vi "Initialize.vi"(8 "error in (no error)":errorcluster, 9 "transceiver settings":T1, 10 "Transfer Groups Configurations":T2[](array[typedef]) {"Transfers"."channel configurations"."buffer offset" format="%d bytes"}, 11 "UDP Transceiver in":refnum<class "UDP Transceiver.lvclass">) -> (0 "error out":errorcluster, 3 "UDP Transceiver out":refnum<class "UDP Transceiver.lvclass">)   [LabVIEW 2017, in "UDP.lvlib" / "UDP Transceiver.lvclass"]
uses:
  UDP Transceiver.lvclass
  Builds/Data Sharing Framework/Current/Data Sharing Framework Core/DSF Core.lvlibp/Configuration/Public/Controls/DSF Engine Transfer Group Configuration.ctl
  Builds/Data Sharing Framework/Current/Data Sharing Framework Core/DSF Core.lvlibp/Configuration/Public/Controls/DSF Direction.ctl
  Builds/Data Sharing Framework/Current/Data Sharing Framework Core/DSF Core.lvlibp/Configuration/Public/Controls/DSF Timing Info.ctl
  Builds/Data Sharing Framework/Current/Data Sharing Framework Core/DSF Core.lvlibp/Configuration/Public/Controls/DSF Engine Transfer Configuration.ctl
  Builds/Data Sharing Framework/Current/Data Sharing Framework Core/DSF Core.lvlibp/Configuration/Public/Controls/DSF Byte Order.ctl
  Builds/Data Sharing Framework/Current/Data Sharing Framework Core/DSF Core.lvlibp/Configuration/Public/Controls/DSF Engine Channel Configuration.ctl
  Builds/Data Sharing Framework/Current/Data Sharing Framework Core/DSF Core.lvlibp/Configuration/Public/Controls/DSF Data Type.ctl
  Builds/Data Sharing Framework/Current/Data Sharing Framework Core/DSF Core.lvlibp/Configuration/Public/Controls/DSF Settings Info.ctl
  UDP Transceiver.lvclass/UDP Transceiver.ctl
  Builds/Data Sharing Framework/Current/Data Sharing Framework Core/DSF Core.lvlibp
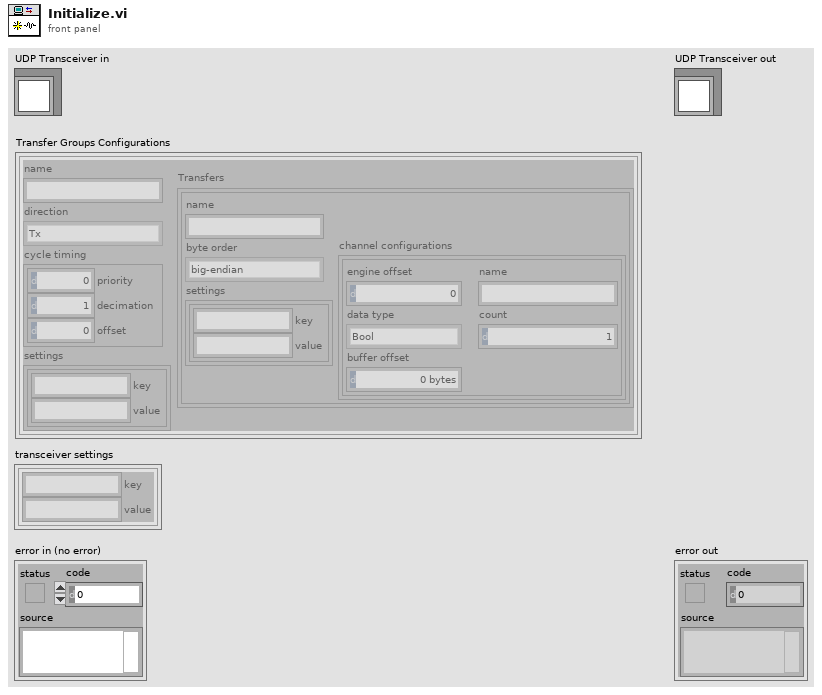
[diagram p1: front panel]
types:
  T1 = typedef "DSF Core.lvlibp/DSF Settings Info.ctl" = cluster{"key":string, "value":string}[]
  T2 = typedef "DSF Core.lvlibp/DSF Engine Transfer Group Configuration.ctl" = cluster{"name":string, "direction":T3, "cycle timing":T4, "Transfers":T5[], "settings":T1}
  T3 = typedef "DSF Core.lvlibp/DSF Direction.ctl" = enum8{"Tx", "Rx"}
  T4 = typedef "DSF Core.lvlibp/DSF Timing Info.ctl" = cluster{"priority":u64, "decimation":u64, "offset":u64}
  T5 = typedef "DSF Core.lvlibp/DSF Engine Transfer Configuration.ctl" = cluster{"name":string, "byte order":T6, "channel configurations":T7[], "settings":T1}
  T6 = typedef "DSF Core.lvlibp/DSF Byte Order.ctl" = enum8{"big-endian", "little-endian"}
  T7 = typedef "DSF Core.lvlibp/DSF Engine Channel Configuration.ctl" = cluster{"engine offset":u64, "name":string, "data type":T8, "count":u64, "buffer offset":u64}
  T8 = typedef "DSF Core.lvlibp/DSF Data Type.ctl" = enum8{"Bool", "SGL", "DBL", "I8", "I16", "I32", "I64", "U8", "U16", "U32", "U64"}
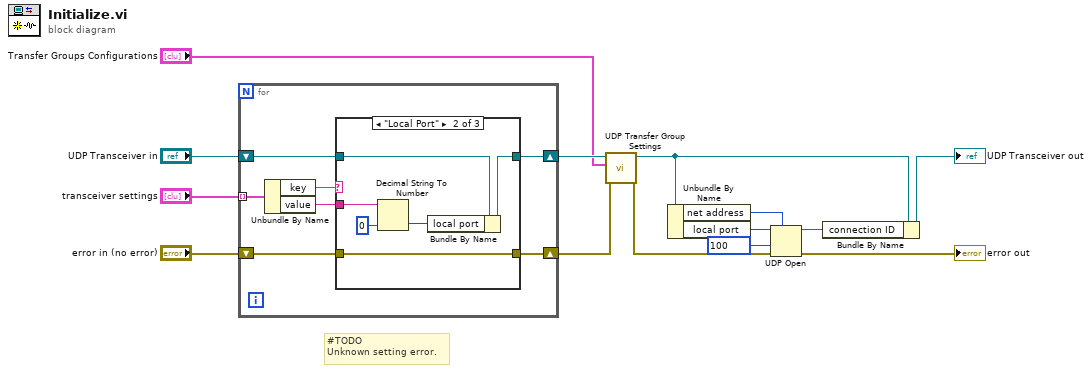
[diagram p0: block diagram]
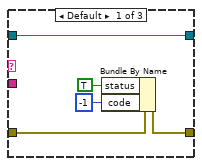
[diagram p2: hidden frame]
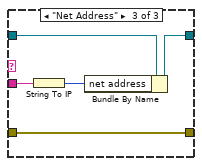
[diagram p3: hidden frame]
diagram:
  # "#TODO\nUnknown setting error."
  n1 = for {
    tunnel: "transceiver settings" -> [w21] mode=indexing
    shift-right: [w17] -> w14
    shift-left: "UDP Transceiver in" -> [w18]
    shift-right: [w15] -> w13
    shift-left: "error in (no error)" -> [w16]
    n2 = Unbundle By Name(w21) -> ("key"=w20:string, "value"=w19:string)
    n3 = case shown="\"Local Port\"" w20 {
      tunnel: w19 -> [_ w31 w34]
      tunnel: w18 -> [w26 w30 w37]
      tunnel: [w26 w29 w36] -> w17
      tunnel: w16 -> [w25 w28 w35]
      tunnel: [w24 w28 w35] -> w15
      frame Default {
        n4 = Bundle By Name(cluster=w25, "status"=TRUE, "code"=-1) -> (w24:errorcluster)
      }
      frame "Local Port" {
        n5 = Decimal String To Number(string=w31, default (0L)=u16 0 ("default (0 I32)")) -> (number=w27:u16)  [unwired: 1 in, 1 out]
        n6 = Bundle By Name(cluster=w30, "local port"=w27) -> (w29:refnum<class "UDP Transceiver.lvclass">)
      }
      frame "Net Address" {
        n7 = String To IP(1:w34) -> (0:w33:u32)
        n8 = Bundle By Name(cluster=w37, "net address"=w33) -> (w36:refnum<class "UDP Transceiver.lvclass">)
      }
    }
  }
  n9 = call "UDP Transfer Group Settings.vi"("error in (no error)"=w13, "Transfer Group Configurations"="Transfer Groups Configurations", "UDP Transceiver in"=w14) -> ("error out"=w12:errorcluster, "UDP Transceiver out"=w11:refnum<class "UDP Transceiver.lvclass">)  [unwired: 7 in]
  n10 = Unbundle By Name(w11) -> ("net address"=w7:u32, "local port"=w10:u16)
  n11 = UDP Open(7:w7, 8:w12, 9:100 ("timeout ms (25000)"), 11:w10) -> (port=w8:refnum<k16>, 0:→"error out":errorcluster)  [unwired: 1 in, 1 out]
  n12 = Bundle By Name(cluster=w11, "connection ID"=w8) -> (→"UDP Transceiver out":refnum<class "UDP Transceiver.lvclass">)
